vi "Encoder.vi"(8 "error in":errorcluster, 11 "Orginal Data":string[][](array[string])) -> (0 "error Out":errorcluster, 3 "Encoded Data":string[][](array[string]))   [LabVIEW 2022 SP3]
uses:
  <vilib>/Utility/file.llb/Read Delimited Spreadsheet (string).vi
  <vilib>/Utility/file.llb/Write Delimited Spreadsheet (string).vi
panel:
  in  "file path (dialog if empty)":path
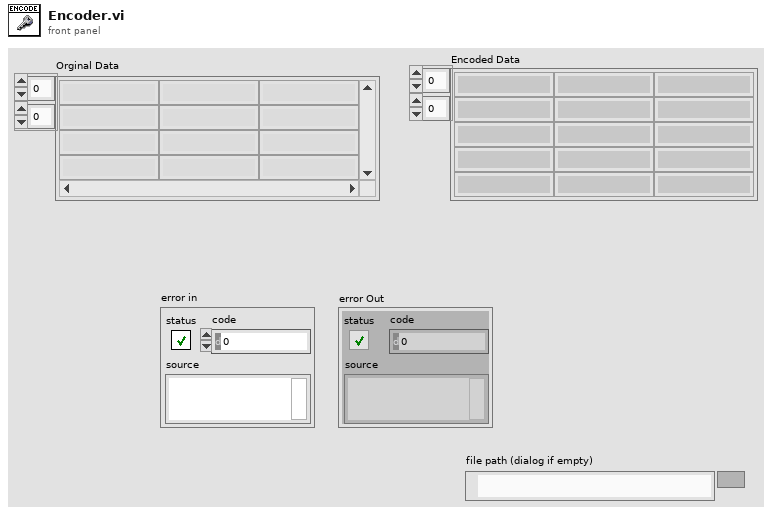
[diagram p1: front panel]
types:
  T1 = cluster{"unsigned byte array[0]":u8, "unsigned byte array[1]":u8, "unsigned byte array[2]":u8}
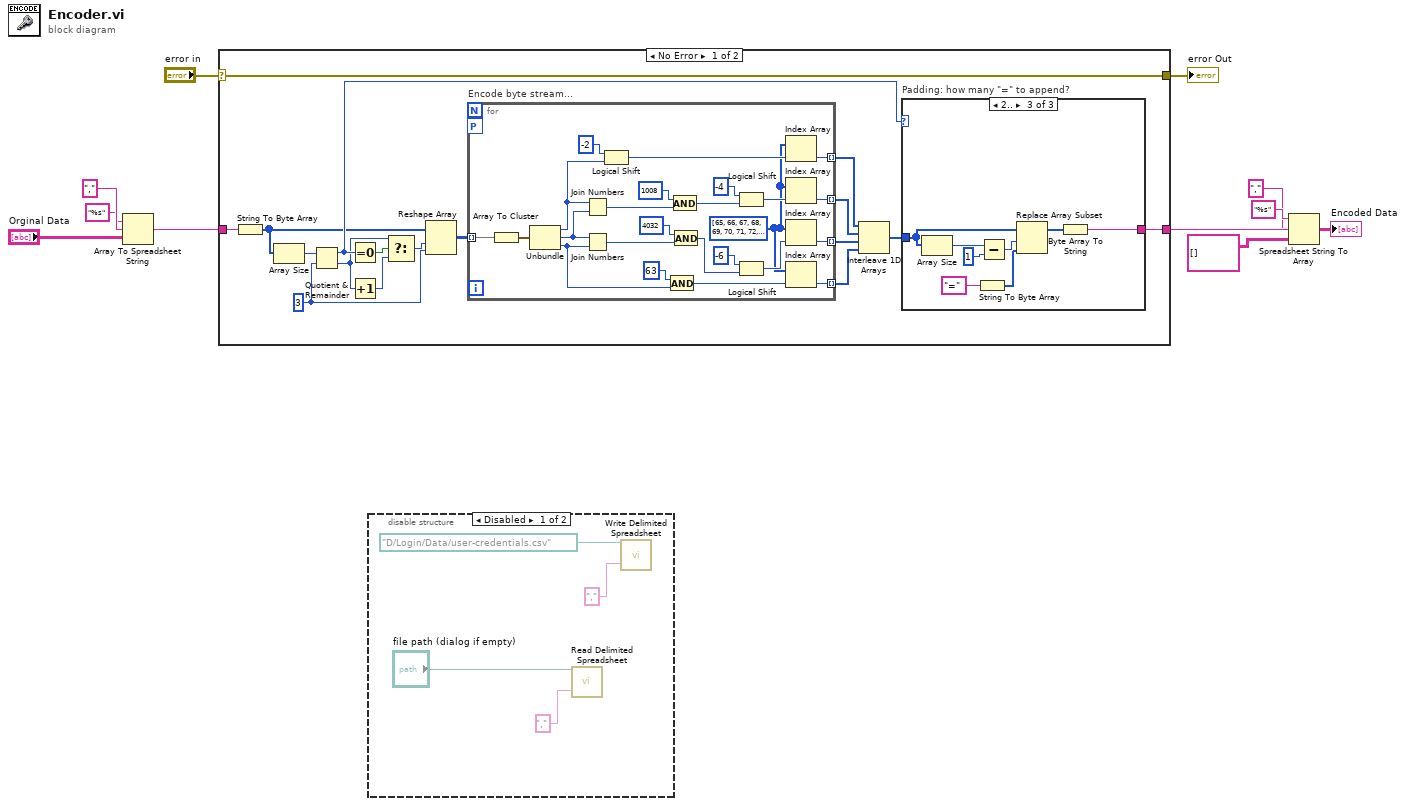
[diagram p0: block diagram]
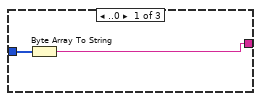
[diagram p3: hidden frame]
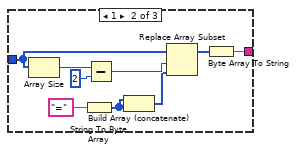
[diagram p4: hidden frame]
diagram:
  n1 = Array To Spreadsheet String(delimiter (Tab)=",", array="Orginal Data", 3:"%s" ("format string")) -> (spreadsheet string=w7:string)
  n2 = case shown="No Error" "error in" {
    selector: "error in" -> [w28 w73]
    tunnel: w7 -> [w14 w72]
    tunnel: [w28 w73] -> w3
    tunnel: [w13 w72] -> w10
    frame No Error {
      w17 = 3 ("y")
      n3 = String To Byte Array(string=w14) -> (unsigned byte array=w18:u8[])
      n4 = Array Size(array=w18) -> (size(s)=w12:i32)
      n5 = Quotient & Remainder(x=w12, y=w17) -> (x-y*floor(x/y)=w26:i32, floor(x/y)=w20:i32)
      n6 = Equal To 0?(x=w26) -> (x = 0?=w27:bool)
      n7 = Increment(x=w20) -> (x+1=w21:i32)
      n8 = Select(t=w20, s=w27, f=w21) -> (s? t:f=w16:i32)
      n9 = Reshape Array(w18, w16, w17) -> (w15:u8[][])
      n10 = for "Encode byte stream..." {
        tunnel: [w31] -> w22 mode=indexing
        tunnel: [w32] -> w23 mode=indexing
        tunnel: [w33] -> w24 mode=indexing
        tunnel: [w34] -> w25 mode=indexing
        workers-P: _ -> [_]
        tunnel: w15 -> [w29] mode=indexing
        w30 = u8[] [65, 66, 67, 68, 69, 70, 71, 72, 73, 74, 75, 76, 77, 78, 79, 80, 81, 82, 83, 84, 85, 86, 87, 88, 89, 90, 97, 98, 99, 100, 101, 102, 103, 104, 105, 106, 107, 108, 109, 110, 111, 112, 113, 114, 115, 116, 117, 118, 119, 120, 121, 122, 48, 49, 50, 51, 52, 53, 54, 55, 56, 57, 43, 47] ("unsigned byte array")
        n11 = Array To Cluster(array=w29) -> (cluster=w52:T1)
        n12 = Unbundle(w52) -> ("unsigned byte array[0]"=w41:u8, "unsigned byte array[1]"=w46:u8, "unsigned byte array[2]"=w40:u8)
        n13 = Join Numbers(hi=w41, lo=w46) -> ((hi.lo)=w50:u16)
        n14 = Join Numbers(hi=w46, lo=w40) -> ((hi.lo)=w45:u16)
        n15 = Logical Shift(y=i8 -2, x=w41) -> (x << y=w38:u8)
        n16 = And(x=u8 63, y=w40) -> (x .and. y?=w35:u8)
        n17 = And(x=u16 1008, y=w50) -> (x .and. y?=w48:u16)
        n18 = And(x=u16 4032, y=w45) -> (x .and. y?=w43:u16)
        n19 = Logical Shift(y=i8 -4, x=w48) -> (x << y=w37:u16)
        n20 = Logical Shift(y=i8 -6, x=w43) -> (x << y=w36:u16)
        n21 = Index Array(array=w30, index=w38) -> (element=w34:u8)
        n22 = Index Array(array=w30, index=w37) -> (element=w33:u8)
        n23 = Index Array(array=w30, index=w36) -> (element=w32:u8)
        n24 = Index Array(array=w30, index=w35) -> (element=w31:u8)
      }
      n25 = Interleave 1D Arrays(w25, w24, w23, w22) -> (w19:u8[])
      n26 = case "Padding: how many \"=\" to append?" shown="2.." w26 {
        tunnel: [w53 w60 w68] -> w13
        tunnel: w19 -> [w54 w58 w66]
        frame ..0 {
          n27 = Byte Array To String(unsigned byte array=w54) -> (string=w53:string)
        }
        frame 1 {
          n28 = Array Size(array=w58) -> (size(s)=w59:i32)
          n29 = String To Byte Array(string="=") -> (unsigned byte array=w56:u8[])
          n30 = Subtract(x=w59, y=2) -> (x-y=w62:i32)
          n31 = Build Array (concatenate)(w56, w56) -> (w55:u8[])
          n32 = Replace Array Subset(array=w58, new element=w55, index=w62) -> (w61:u8[])
          n33 = Byte Array To String(unsigned byte array=w61) -> (string=w60:string)
        }
        frame 2.. {
          n34 = Array Size(array=w66) -> (size(s)=w67:i32)
          n35 = String To Byte Array(string="=") -> (unsigned byte array=w64:u8[])
          n36 = Subtract(x=w67, y=1) -> (x-y=w70:i32)
          n37 = Replace Array Subset(array=w66, new element=w64, index=w70) -> (w69:u8[])
          n38 = Byte Array To String(unsigned byte array=w69) -> (string=w68:string)
        }
      }
    }
    frame Error {
    }
  }
  "error Out" <- w3
  n39 = disable-structure shown="Disabled" {
    frame Disabled {
      n40 = call-poly <vilib>:"Read Delimited Spreadsheet.vi"("file path (dialog if empty)"="file path (dialog if empty)", "delimiter (\\t)"="," ("delimiter (\\t)")) -> ()  [unwired: 8 in, 6 out]
      n41 = call-poly <vilib>:"Write Delimited Spreadsheet.vi"("file path (dialog if empty)"=path "D:/Login/Data/user-credentials.csv", "delimiter (\\t)"="," ("delimiter (\\t)")) -> ()  [unwired: 12 in, 2 out]
    }
    frame Enabled {
    }
  }
  n42 = Spreadsheet String To Array(delimiter (Tab)=",", format string="%s", spreadsheet string=w10, array type (2D Dbl)=string[][] [] ("all rows")) -> (array=→"Encoded Data":string[][])
